vi "Ic readout_clocked_dist V2.vi"() -> ()   [LabVIEW 2023]
uses:
  <vilib>/LabVIEW Targets/FPGA/cRIO/shared/nicrio_ModuleControls/nicrio_cRIO-9775_TriggerSlope.ctl
  <vilib>/LabVIEW Targets/FPGA/cRIO/shared/nicrio_ModuleControls/nicrio_BasicConversionTime.ctl
  <vilib>/LabVIEW Targets/FPGA/cRIO/shared/nicrio_ModuleControls/nicrio_cRIO-9775_RecordDataRates4ChansRing.ctl
  <vilib>/rvi/Emulation/niFpgaGetClockAttributes.vi
  <vilib>/rvi/Emulation/niFpgaSctlEmulationGetInTimedLoop.vi
  <vilib>/rvi/Emulation/niFpgaEmulationReportErrorSimple.vi
  <vilib>/rvi/Emulation/niFpgaProcessEmulError.vi
  <vilib>/rvi/Emulation/niFpgaCriticalErrorInLSC.vi
  <vilib>/rvi/eio/common/nirviEmuTemplateMethod_errors.vi
  <vilib>/rvi/eio/common/nirviEmuTemplatePropertySet_errors.vi
  <vilib>/eio/utilities/niEioResolveVilibRelativePath.vi
  <vilib>/rvi/interface/RandomDataEmulation/niFpgaRandomDataHandleErrors.vi
  <vilib>/eio/EIOMethodNode/EIOMethodNode.xnode
  <vilib>/eio/EIONode/EIONode.xnode
  <vilib>/eio/EIOPropertyNode/EIOPropertyNode.xnode
  <vilib>/rvi/DataTransferAndStorage/Container/XNode/niFpgaContainer.xnode
  <vilib>/rvi/interface/RandomDataEmulation/nirviRandomDataFpgaReadWriteTemplate.vi
  <vilib>/rvi/eio/common/nirviEmuTemplatePropertyGet_errors.vi
  <vilib>/rvi/eio/common/nirviEmuTemplatePropertyGet_noerrors.vi
  <vilib>/rvi/eio/common/nirviEmuTemplatePropertySet_noerrors.vi
panel:
  in  "Count ms":u32=20
  out "Clock":bool
  in  "stop":bool
  in  "Gate wait time us":u32=100
  in  "Ic Cut off or curve":bool
  in  "Timeout":i32=-1
  in  "Record Samples":u32=25
  in  "Record PreTrigger Samples":u32=1
  in  "Record Data Rate":T1=1 items=["20.000 MS/s (NI 9775)"=1, "10.00 MS/s (NI 9775)"=2, "6.667 MS/s (NI 9775)"=3, "5.000 MS/s (NI 9775)"=4, "2.500 MS/s (NI 9775)"=8, "1.667 MS/s (NI 9775)"=12, "1.250 MS/s (NI 9775)"=16, "1.000 MS/s (NI 9775)"=20, "833.333 KS/s (NI 9775)"=24, "714.286 KS/s (NI 9775)"=28, "625.000 KS/s (NI 9775)"=32, "555.556 KS/s (NI 9775)"=36, "500.000 KS/s (NI 9775)"=40, "454.545 KS/s (NI 9775)"=44, "416.667 KS/s (NI 9775)"=48, "384.615 KS/s (NI 9775)"=52, "357.143 KS/s (NI 9775)"=56, "333.333 KS/s (NI 9775)"=60, "312.500 KS/s (NI 9775)"=64, "294.118 KS/s (NI 9775)"=68, "277.778 KS/s (NI 9775)"=72, "263.158 KS/s (NI 9775)"=76, "250.000 KS/s (NI 9775)"=80, "238.095 KS/s (NI 9775)"=84, "227.273 KS/s (NI 9775)"=88, "217.391 KS/s (NI 9775)"=92, "208.333 KS/s (NI 9775)"=96, "200.000 KS/s (NI 9775)"=100, "192.308 KS/s (NI 9775)"=104, "185.185 KS/s (NI 9775)"=108, "178.571 KS/s (NI 9775)"=112, "172.414 KS/s (NI 9775)"=116, "166.667 KS/s (NI 9775)"=120, "161.290 KS/s (NI 9775)"=124, "156.250 KS/s (NI 9775)"=128, "151.515 KS/s (NI 9775)"=132, "147.059 KS/s (NI 9775)"=136, "142.857 KS/s (NI 9775)"=140, "138.889 KS/s (NI 9775)"=144, "135.135 KS/s (NI 9775)"=148, "131.579 KS/s (NI 9775)"=152, "128.205 KS/s (NI 9775)"=156, "125.000 KS/s (NI 9775)"=160, "121.951 KS/s (NI 9775)"=164, "119.048 KS/s (NI 9775)"=168, "116.279 KS/s (NI 9775)"=172, "113.636 KS/s (NI 9775)"=176, "111.111 KS/s (NI 9775)"=180, "108.696 KS/s (NI 9775)"=184, "106.383 KS/s (NI 9775)"=188, "104.167 KS/s (NI 9775)"=192, "102.041 KS/s (NI 9775)"=196, "100.000 KS/s (NI 9775)"=200, "50.000 KS/s (NI 9775)"=400, "33.333 KS/s (NI 9775)"=600, "25.000 KS/s (NI 9775)"=800, "20.000 KS/s (NI 9775)"=1000, "16.667 KS/s (NI 9775)"=1200, "14.286 KS/s (NI 9775)"=1400, "12.500 KS/s (NI 9775)"=1600, "11.111 KS/s (NI 9775)"=1800, "10.000 KS/s (NI 9775)"=2000, "9.091 KS/s (NI 9775)"=2200, "8.333 KS/s (NI 9775)"=2400, "7.692 KS/s (NI 9775)"=2600, "7.143 KS/s (NI 9775)"=2800, "6.667 KS/s (NI 9775)"=3000, "6.250 KS/s (NI 9775)"=3200, "5.882 KS/s (NI 9775)"=3400, "5.556 KS/s (NI 9775)"=3600, "5.000 KS/s (NI 9775)"=4000, "4.762 KS/s (NI 9775)"=4200, "4.545 KS/s (NI 9775)"=4400, "4.348 KS/s (NI 9775)"=4600, "4.167 KS/s (NI 9775)"=4800, "4.000 KS/s (NI 9775)"=5000, "3.846 KS/s (NI 9775)"=5200, "3.571 KS/s (NI 9775)"=5600, "3.333 KS/s (NI 9775)"=6000, "3.125 KS/s (NI 9775)"=6400, "2.941 KS/s (NI 9775)"=6800, "2.778 KS/s (NI 9775)"=7200, "2.632 KS/s (NI 9775)"=7600, "2.500 KS/s (NI 9775)"=8000, "2.381 KS/s (NI 9775)"=8400, "2.273 KS/s (NI 9775)"=8800, "2.174 KS/s (NI 9775)"=9200, "2.083 KS/s (NI 9775)"=9600, "2.000 KS/s (NI 9775)"=10000, "1.923 KS/s (NI 9775)"=10400, "1.852 KS/s (NI 9775)"=10800, "1.786 KS/s (NI 9775)"=11200, "1.724 KS/s (NI 9775)"=11600, "1.667 KS/s (NI 9775)"=12000, "1.613 KS/s (NI 9775)"=12400, "1.563 KS/s (NI 9775)"=12800, "1.515 KS/s (NI 9775)"=13200, "1.471 KS/s (NI 9775)"=13600, "1.429 KS/s (NI 9775)"=14000, "1.389 KS/s (NI 9775)"=14400, "1.351 KS/s (NI 9775)"=14800, "1.316 KS/s (NI 9775)"=15200, "1.282 KS/s (NI 9775)"=15600, "1.250 KS/s (NI 9775)"=16000, "1.220 KS/s (NI 9775)"=16400, "1.190 KS/s (NI 9775)"=16800, "1.163 KS/s (NI 9775)"=17200, "1.136 KS/s (NI 9775)"=17600, "1.111 KS/s (NI 9775)"=18000, "1.087 KS/s (NI 9775)"=18400, "1.064 KS/s (NI 9775)"=18800, "1.042 KS/s (NI 9775)"=19200, "1.020 KS/s (NI 9775)"=19600, "1.000 KS/s (NI 9775)"=20000, "0.980 KS/s (NI 9775)"=20400, "0.962 KS/s (NI 9775)"=20800, "0.943 KS/s (NI 9775)"=21200, "0.926 KS/s (NI 9775)"=21600, "0.909 KS/s (NI 9775)"=22000, "0.893 KS/s (NI 9775)"=22400, "0.877 KS/s (NI 9775)"=22800, "0.862 KS/s (NI 9775)"=23200, "0.847 KS/s (NI 9775)"=23600, "0.833 KS/s (NI 9775)"=24000, "0.820 KS/s (NI 9775)"=24400, "0.806 KS/s (NI 9775)"=24800, "0.794 KS/s (NI 9775)"=25200, "0.781 KS/s (NI 9775)"=25600, "0.694 KS/s (NI 9775)"=28800, "0.625 KS/s (NI 9775)"=32000, "0.568 KS/s (NI 9775)"=35200, "0.521 KS/s (NI 9775)"=38400, "0.446 KS/s (NI 9775)"=44800, "0.391 KS/s (NI 9775)"=51200, "0.347 KS/s (NI 9775)"=57600, "0.313 KS/s (NI 9775)"=64000]
  in  "Timing Mode":T2
  in  "Records Num":i32=1
  in  "AI Trigger Configuration":T4={"Trigger Slope"=enum."Positive", "Trigger Level"=1.199951171875, "Hystesis Value"=1.10009765625, "AI Channel"=0}
  out "error out":errorcluster
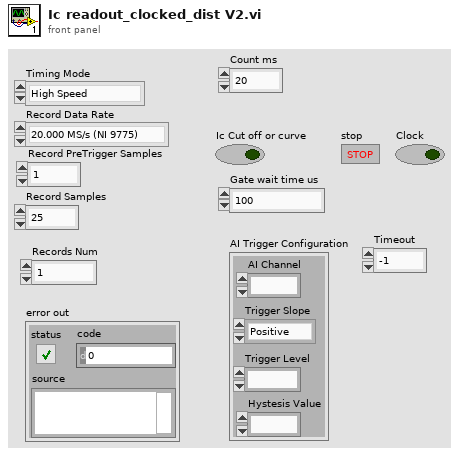
[diagram p1: front panel]
types:
  T1 = typedef "nicrio_cRIO-9775_RecordDataRates4ChansRing.ctl" = u16
  T2 = typedef "nicrio_BasicConversionTime.ctl" = enum8{"High Speed", "High Resolution"}
  T3 = typedef "nicrio_cRIO-9775_TriggerSlope.ctl" = enum8{"Positive", "Negative"}
  T4 = cluster{"Trigger Slope":T3, "Trigger Level":fxp<+/-,17,5>, "Hystesis Value":fxp<+,16,4>, "AI Channel":u8}
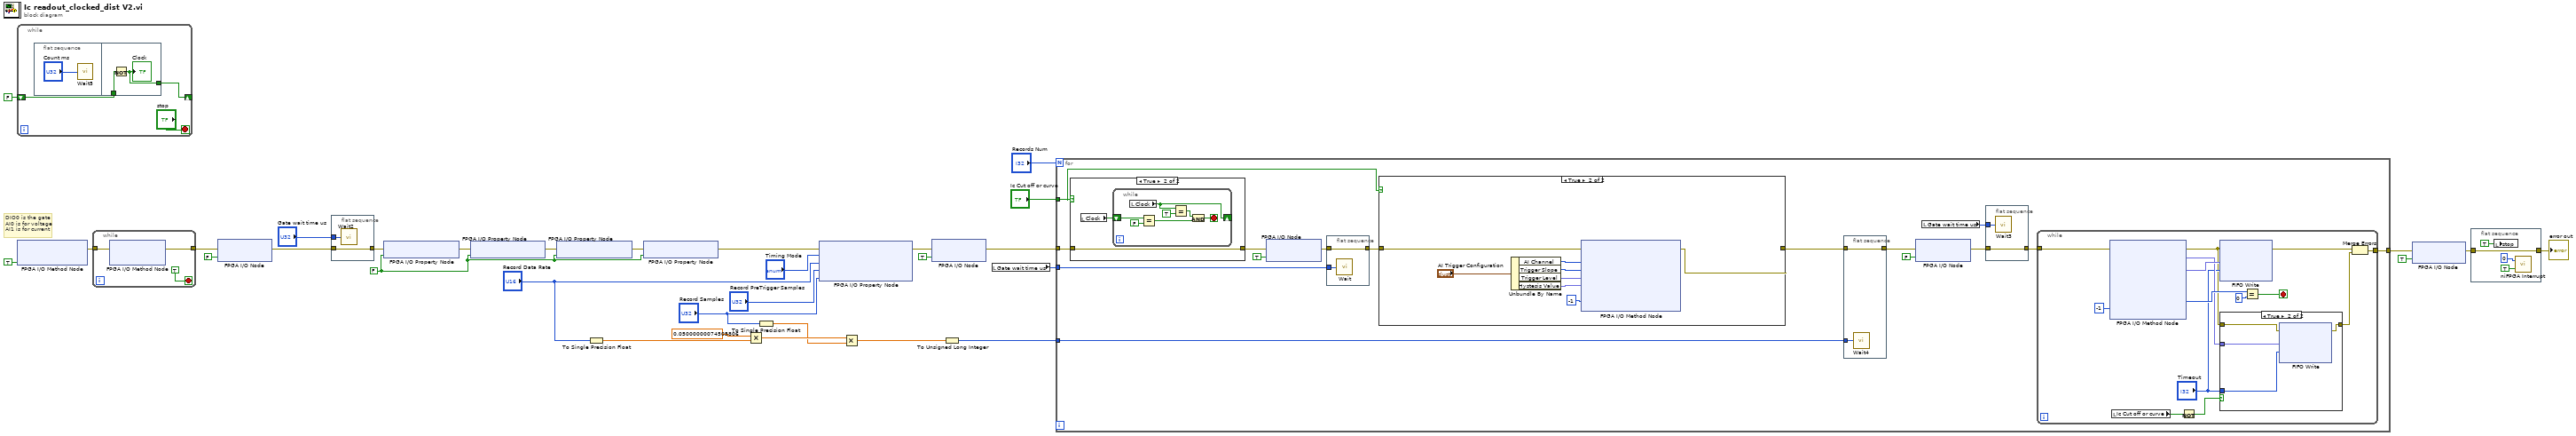
[diagram p0: block diagram]
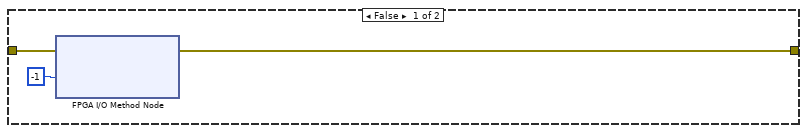
[diagram p3: hidden frame]
diagram:
  w24 = FALSE ("Enable Low Pass Filter")
  # "DIO0 is the gate\nAI0 is for voltage\nAI1 is for current"
  n1 = while {
    shift-right: [w34] -> _
    shift-left: FALSE ("Clock") -> [w35]
    stop <- "stop" stop-if-true
    n2 = flat-sequence {
      tunnel: w35 -> [w39]
      tunnel: [w38] -> w34
      frame #0 {
        n3 = call "Wait5"("Count(mSec)"="Count ms") -> ()  [unwired: 1 out]
      }
      frame #1 {
        n4 = Not(x=w39) -> (.not. x?=w38:bool)
        "Clock" <- w38
      }
    }
  }
  n5 = xnode "FPGA I/O Method Node"("Enable"=TRUE) -> ("error out"=w29:errorcluster)  [unwired: 2 in, 1 out]
  n6 = while {
    tunnel: w29 -> [w42]
    tunnel: [w41] -> w28
    stop <- TRUE stop-if-true
    n7 = xnode "FPGA I/O Method Node"("error in"=w42) -> ("error out"=w41:errorcluster)  [unwired: 1 in, 2 out]
  }
  n8 = xnode "FPGA I/O Node"("error in"=w28, "Mod2/DIO0"=FALSE) -> ("error out"=w17:errorcluster)  [unwired: 1 in, 1 out]
  n9 = flat-sequence {
    tunnel: w17 -> [w44]
    tunnel: [w44] -> w16
    tunnel: "Gate wait time us" -> [w43]
    frame #0 {
      n10 = call "Wait2"("Count(uSec)"=w43) -> ()  [unwired: 1 out]
    }
  }
  n11 = xnode "FPGA I/O Property Node"("error in"=w16, "Enable Analog Filter"=w24) -> ("error out"=w27:errorcluster)  [unwired: 1 in, 1 out]
  n12 = xnode "FPGA I/O Property Node"("error in"=w27, "Enable Analog Filter"=w24) -> ("error out"=w26:errorcluster)  [unwired: 1 in, 1 out]
  n13 = xnode "FPGA I/O Property Node"("error in"=w26, "Enable Analog Filter"=w24) -> ("error out"=w25:errorcluster)  [unwired: 1 in, 1 out]
  n14 = To Single Precision Float(number="Record Data Rate") -> (single precision float=w8:sgl)
  n15 = xnode "FPGA I/O Property Node"("error in"=w25, "Enable Analog Filter"=w24) -> ("error out"=w23:errorcluster)  [unwired: 1 in, 1 out]
  n16 = Multiply(x=sgl 0.05, y=w8) -> (x*y=w7:sgl)
  n17 = To Single Precision Float(number="Record Samples") -> (single precision float=w5:sgl)
  n18 = xnode "FPGA I/O Property Node"("error in"=w23, "Timing Mode"="Timing Mode", "Record Data Rate"="Record Data Rate", "Record PreTrigger Samples"="Record PreTrigger Samples", "Record Samples"="Record Samples") -> ("error out"=w22:errorcluster)  [unwired: 1 in, 1 out]
  n19 = Multiply(x=w7, y=w5) -> (x*y=w4:sgl)
  n20 = xnode "FPGA I/O Node"("error in"=w22, "Mod1/Start"=TRUE) -> ("error out"=w2:errorcluster)  [unwired: 1 in, 1 out]
  n21 = To Unsigned Long Integer(number=w4) -> (unsigned 32bit integer=w3:u32)
  n22 = local read "Gate wait time us"() -> (w13:u32)
  n23 = for {
    N: "Records Num" -> [_]
    tunnel: w2 -> [w46]
    tunnel: "Ic Cut off or curve" -> [w47]
    tunnel: [w57] -> w14
    tunnel: w13 -> [w56]
    tunnel: w3 -> [w48]
    n24 = case shown="True" w47 {
      tunnel: w46 -> [w60 w62]
      tunnel: [w60 w62] -> w45
      frame False {
      }
      frame True {
        n25 = local read "Clock"() -> (w61:bool)
        n26 = while {
          shift-right: [w64] -> _
          shift-left: w61 -> [w68]
          stop <- w63 stop-if-true
          n27 = local read "Clock"() -> (w64:bool)
          n28 = Equal?(x=w68, y=FALSE) -> (x = y?=w65:bool)
          n29 = Equal?(x=w64, y=TRUE) -> (x = y?=w66:bool)
          n30 = And(x=w66, y=w65) -> (x .and. y?=w63:bool)
        }
      }
    }
    n31 = xnode "FPGA I/O Node"("error in"=w45, "Mod2/DIO0"=TRUE) -> ("error out"=w55:errorcluster)  [unwired: 1 in, 1 out]
    n32 = flat-sequence {
      tunnel: w56 -> [w75]
      tunnel: w55 -> [w74]
      tunnel: [w74] -> w54
      frame #0 {
        n33 = call "Wait"("Count(uSec)"=w75) -> ()  [unwired: 1 out]
      }
    }
    n34 = case shown="True" w47 {
      tunnel: w54 -> [w77 w86]
      tunnel: [w76 w79] -> w50
      frame False {
        n35 = xnode "FPGA I/O Method Node"("error in"=w77, "Timeout (Ticks)"=-1) -> ("error out"=w76:errorcluster)  [unwired: 1 in, 2 out]
      }
      frame True {
        n36 = Unbundle By Name("AI Trigger Configuration") -> ("AI Channel"=w85:u8, "Trigger Slope"=w84:T3, "Trigger Level"=w83:fxp<+/-,17,5>, "Hystesis Value"=w82:fxp<+,16,4>)
        n37 = xnode "FPGA I/O Method Node"("error in"=w86, "AI Channel"=w85, "Trigger Slope"=w84, "Trigger Level"=w83, "Hysteresis Value"=w82, "Timeout (Ticks)"=-1) -> ("error out"=w79:errorcluster)  [unwired: 1 in, 3 out]
      }
    }
    n38 = flat-sequence {
      tunnel: w50 -> [w71]
      tunnel: [w71] -> w49
      tunnel: w48 -> [w70]
      frame #0 {
        n39 = call "Wait4"("Count(uSec)"=w70) -> ()  [unwired: 1 out]
      }
    }
    n40 = xnode "FPGA I/O Node"("error in"=w49, "Mod2/DIO0"=FALSE) -> ("error out"=w53:errorcluster)  [unwired: 1 in, 1 out]
    n41 = local read "Gate wait time us"() -> (w52:u32)
    n42 = flat-sequence {
      tunnel: w52 -> [w73]
      tunnel: w53 -> [w72]
      tunnel: [w72] -> w51
      frame #0 {
        n43 = call "Wait3"("Count(uSec)"=w73) -> ()  [unwired: 1 out]
      }
    }
    n44 = while {
      tunnel: w51 -> [w100]
      tunnel: [w89] -> w57
      stop <- w96 stop-if-true
      n45 = xnode "FPGA I/O Method Node"("error in"=w100, "Timeout (Ticks)"=-1) -> ("error out"=w92:errorcluster, "AI0"=w94:fxp<+/-,17,5>, "AI1"=w95:fxp<+/-,17,5>, "Elements Remaining"=w98:u32)  [unwired: 1 in, 5 out]
      n46 = local read "Ic Cut off or curve"() -> (w88:bool)
      n47 = Not(x=w88) -> (.not. x?=w87:bool)
      n48 = xnode ("FIFO Write")("Element"=w95, "Timeout"="Timeout", "error in (no error)"=w92) -> ("error out"=w91:errorcluster)  [unwired: 1 in, 2 out]
      n49 = case shown="True" w87 {
        tunnel: w94 -> [_ w105]
        tunnel: "Timeout" -> [_ w104]
        tunnel: w92 -> [w101 w103]
        tunnel: [w101 w102] -> w90
        frame False {
        }
        frame True {
          n50 = xnode ("FIFO Write")("Element"=w105, "Timeout"=w104, "error in (no error)"=w103) -> ("error out"=w102:errorcluster)  [unwired: 1 in, 2 out]
        }
      }
      n51 = Equal?(x=w98, y=u32 0) -> (x = y?=w96:bool)
      n52 = Merge Errors(w91, w90) -> (w89:errorcluster)
    }
  }
  n53 = xnode "FPGA I/O Node"("error in"=w14, "Mod1/Stop"=TRUE) -> ("error out"=w12:errorcluster)  [unwired: 1 in, 1 out]
  n54 = flat-sequence {
    tunnel: w12 -> [w109]
    tunnel: [w109] -> w11
    frame #0 {
      n55 = local write "stop"(TRUE ("stop")) -> ()
      n56 = call <vilib>:"niFPGA Interrupt.vi"("Wait Until Cleared (F)"=TRUE, "IRQ Number (0)"=u8 0) -> ()  [unwired: 1 in]
    }
  }
  "error out" <- w11
